vi "Read Shift.vi"(8 "error in (no error)":errorcluster, 11 "KeyDown in":refnum<class "KeyDown.lvclass">) -> (0 "error out":errorcluster, 2 "Shift":bool, 3 "KeyDown out":refnum<class "KeyDown.lvclass">)   [LabVIEW 2016, in "DataGrid.lvlib" / "KeyDown.lvclass"]
uses:
  <userlib>/LabVIEWdotNetDataGrid/source/Events/KeyDown/KeyDown.lvclass
  <userlib>/LabVIEWdotNetDataGrid/source/Events/KeyDown/KeyDown.lvclass/KeyDown.ctl
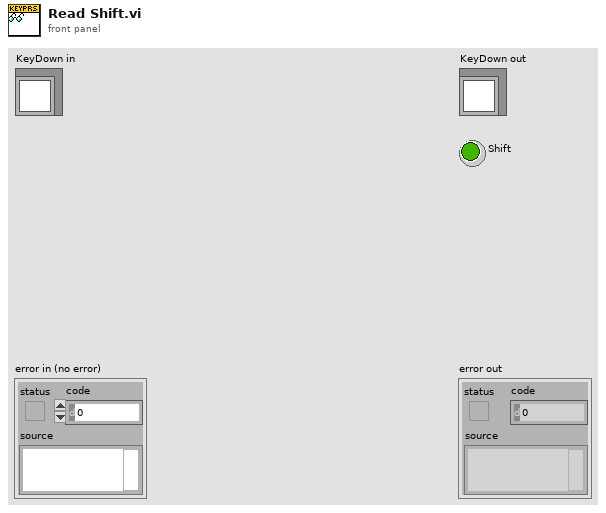
[diagram p1: front panel]
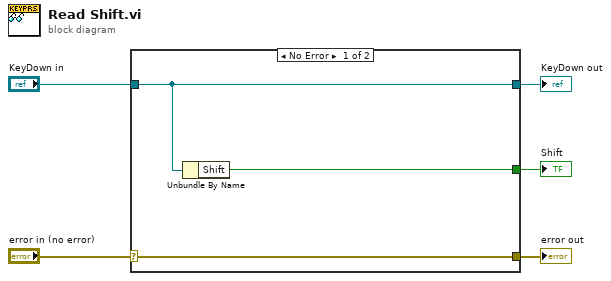
[diagram p0: block diagram]
diagram:
  n1 = case shown="No Error" "error in (no error)" {
    selector: "error in (no error)" -> [w8 w9]
    tunnel: [w8 w9] -> w4
    tunnel: [w7 w10] -> w2
    tunnel: "KeyDown in" -> [w7 w10]
    tunnel: [w6 _] -> w1
    frame No Error {
      n2 = Unbundle By Name(w7) -> ("Shift"=w6:bool)
    }
    frame Error {
    }
  }
  "error out" <- w4
  "KeyDown out" <- w2
  "Shift" <- w1
